vi "send_unavailable.vi"(8 "error in (no error)":errorcluster, 10 "title":string, 11 "client id":refnum<k5>) -> (0 "error out":errorcluster, 3 "client id out":refnum<k5>)   [LabVIEW 2020, in "librarian.lvclass"]
uses:
  librarian.lvclass
  shared/message--cluster.ctl
  shared/request--enum.ctl
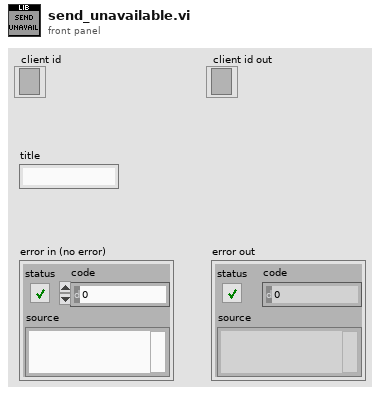
[diagram p1: front panel]
types:
  T1 = typedef "request--enum.ctl" = enum16{"CHECKIN", "CHECKOUT"}
  T2 = typedef "message--cluster.ctl" = cluster{"header":string, "cmd":T1, "title":string, "book":string}
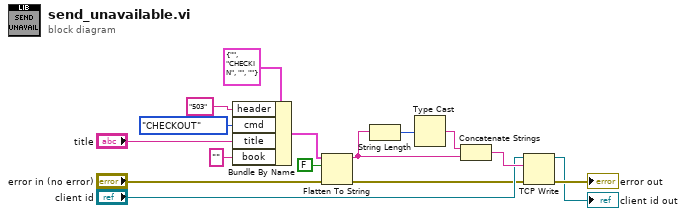
[diagram p0: block diagram]
diagram:
  n1 = Bundle By Name(cluster=T2 {"header"="", "cmd"=enum."CHECKIN", "title"="", "book"=""} ("request"), "header"="503", "cmd"=request--enum."CHECKOUT", "title"="title", "book"="") -> (w13:T2)
  n2 = Flatten To String(anything=w13, prepend array or string size? (T)=FALSE, error in (no error)="error in (no error)") -> (data string=w7:string, error out=w4:errorcluster)  [unwired: 1 in, 1 out]
  n3 = String Length(string=w7) -> (length=w9:i32)
  n4 = Type Cast(x=w9) -> (*(type *) &x=w8:string)  [unwired: 1 in]
  n5 = Concatenate Strings(w8, w7) -> (w6:string)
  n6 = TCP Write(connection ID="client id", data in=w6, error in (no error)=w4) -> (connection ID out=→"client id out":refnum<k5>, error out=→"error out":errorcluster)  [unwired: 2 out]
